vi "setFreqVI.vi"(1 "error in":errorcluster, 2 "Frequenz in Hz":dbl) -> (0 "error out":errorcluster)   [LabVIEW 2010]
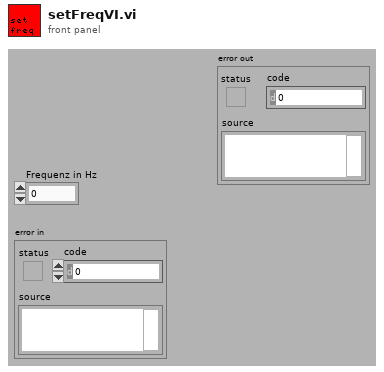
[diagram p1: front panel]
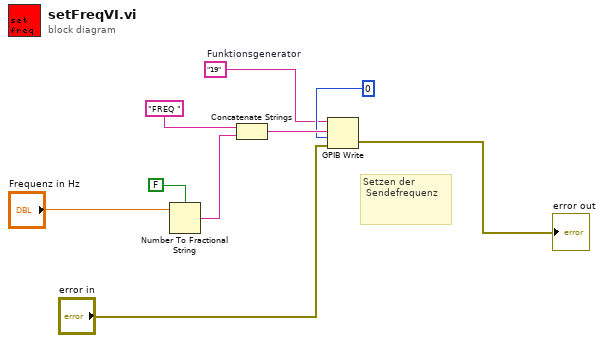
[diagram p0: block diagram]
diagram:
  w2 = "19"  # Funktionsgenerator
  # "Setzen der \n Sendefrequenz"
  n1 = Number To Fractional String(use system decimal point (T)=FALSE, number="Frequenz in Hz") -> (F-format string=w6:string)  [unwired: 2 in]
  n2 = Concatenate Strings("FREQ ", w6) -> (w4:string)
  n3 = GPIB Write(0:w2, 1:w4, 2:i16 0 ("mode (0)"), 3:"error in") -> (6:→"error out":errorcluster)  [unwired: 1 in, 1 out]
